vi "usrp_mimo_ofdm_2x2_freq_MRC.vi"() -> ()   [LabVIEW 2014]
uses:
  <instrlib>/niUSRP/niUSRP Timestamp.ctl
  <vilib>/addons/Modulation/Analog/controls/Complex Data Waveform.ctl
  <vilib>/addons/Modulation/Digital/General/MT Generate Bits (Galois, PN Order).vi
  <vilib>/addons/Modulation/Digital/Support/Common/Validators/mod_Generate Bits Validate.vi
  <vilib>/addons/Modulation/Analog/support/mod_Set Error Source.vi
  <instrlib>/niUSRP/niUSRP Configure Time Start Trigger.vi
  <vilib>/addons/Modulation/Digital/General/MT Generate QAM System Parameters(M).vi
  <vilib>/addons/Modulation/Digital/Support/Common/Validators/mod_Generate Filter Coefficients Validate.vi
  <vilib>/addons/Modulation/Digital/General/subVIs/mod_Generate Filter Coefficients.vi
  <vilib>/addons/Modulation/Digital/General/subVIs/mod_Generate Bits PN Sequence.vi
  <vilib>/addons/Modulation/Digital/General/MT Map Bits to QAM Symbols.vi
  <vilib>/addons/Modulation/Digital/General/MT Apply Pulse Shaping Filter (Generic).vi
  <instrlib>/niUSRP/niUSRP Write Tx Data (2D CDB).vi
  <instrlib>/niUSRP/niUSRP Fetch Rx Data (2D CDB).vi
  <vilib>/addons/Modulation/Digital/General/MT Apply Matched Filter (Generic).vi
  <vilib>/addons/Modulation/Digital/General/MT Align to Ideal Symbols (Generic).vi
  <vilib>/measure/maspectr.llb/FFT Power Spectrum and PSD for 1 Chan (CDB).vi
  <vilib>/addons/Modulation/Digital/General/MT Map QAM Symbols to Bits.vi
  <vilib>/addons/Modulation/niDMT.lvlib
  <vilib>/measure/NI_MAPro.lvlib
  <vilib>/addons/Modulation/niAMT.lvlib
panel:
  out "Decoded Constellation Map":cdb[](graph)
  out "Decoded Constellation Map 2":cdb[](graph)
  out "Waveform Chart":i16(graph)
  out "sum":i16
  out "x = 0?":bool
  out "input bits stream":i8[](array[numeric]) caption="input bit stream"
  out "output bit stream":i8[](array[numeric])
  in  "CP length":u32=32 caption="CP Size"
  in  "Message Carrier":u32=128
  in  "FFT Size":u32=256
  in  "RXa:Timebase Clock Source":string(combo)="Internal"
  in  "RXa:Reference Frequency Source":string(combo)="Internal"
  in  "TXa:Timebase Clock Source":string(combo)="Internal"
  in  "TXa:Reference Frequency Source":string(combo)="Internal"
  out "OFF":bool=TRUE
  out "RX error":bool
  out "TX error":bool
  out "ERROR":bool
  out "Decoded Constellation Map 1":cdb[](graph)
  in  "TX timeout":dbl=10.0
  out "error IO":errorcluster
  in  "stop":bool
  out "Transmitted Constellation Map":cluster{dbl[], dbl[]}[](graph)
  out "PSD of Received Signal":cluster{"f0":dbl, "df":dbl, "magnitude":dbl[]}[](graph)
  out "USRP timestamp":T1={"whole seconds"=11, "fractional seconds"=0.9000012199999999}
  in  "number of samples":i64=100000
  in  "M-QAM (16)":i32=16
  in  "total bits (128)":i32=512 caption="total bits (512)"
  in  "filter length (symbols)":i32=8
  in  "filter parameter":dbl=0.5 format="%.2f"
  in  "samples per symbol (16)":i32=4
  in  "pulse shaping filter (none)":T2(ring)=enum."Raised Cosine"
  in  "RXb:Timebase Clock Source":string(combo)="Mimo"
  in  "RXb:Reference Frequency Source":string(combo)="Mimo"
  in  "TXb:Timebase Clock Source":string(combo)="Mimo"
  in  "TXb:Reference Frequency Source":string(combo)="Mimo"
  in  "RXb Active Antenna":string="RX2"
  in  "TXb Active Antenna":string="TX1"
  in  "RXb Gain":dbl
  in  "TXb Gain":dbl
  in  "RXa Active Antenna":string="RX2"
  in  "RXa Gain":dbl
  in  "TXa Active Antenna":string="TX1"
  in  "TXa Gain":dbl
  in  "Carrier Frequency":dbl=1200000000.0 format="%#_6p"
  in  "IQ Rate":dbl=1000000.0 format="%#_6p"
  in  "TX device names":refnum<k15>="192.168.10.2;192.168.10.5"
  in  "start trigger time":T1={"whole seconds"=4, "fractional seconds"=0.1}
  in  "RX device names":refnum<k15>="192.168.10.2;192.168.10.5"
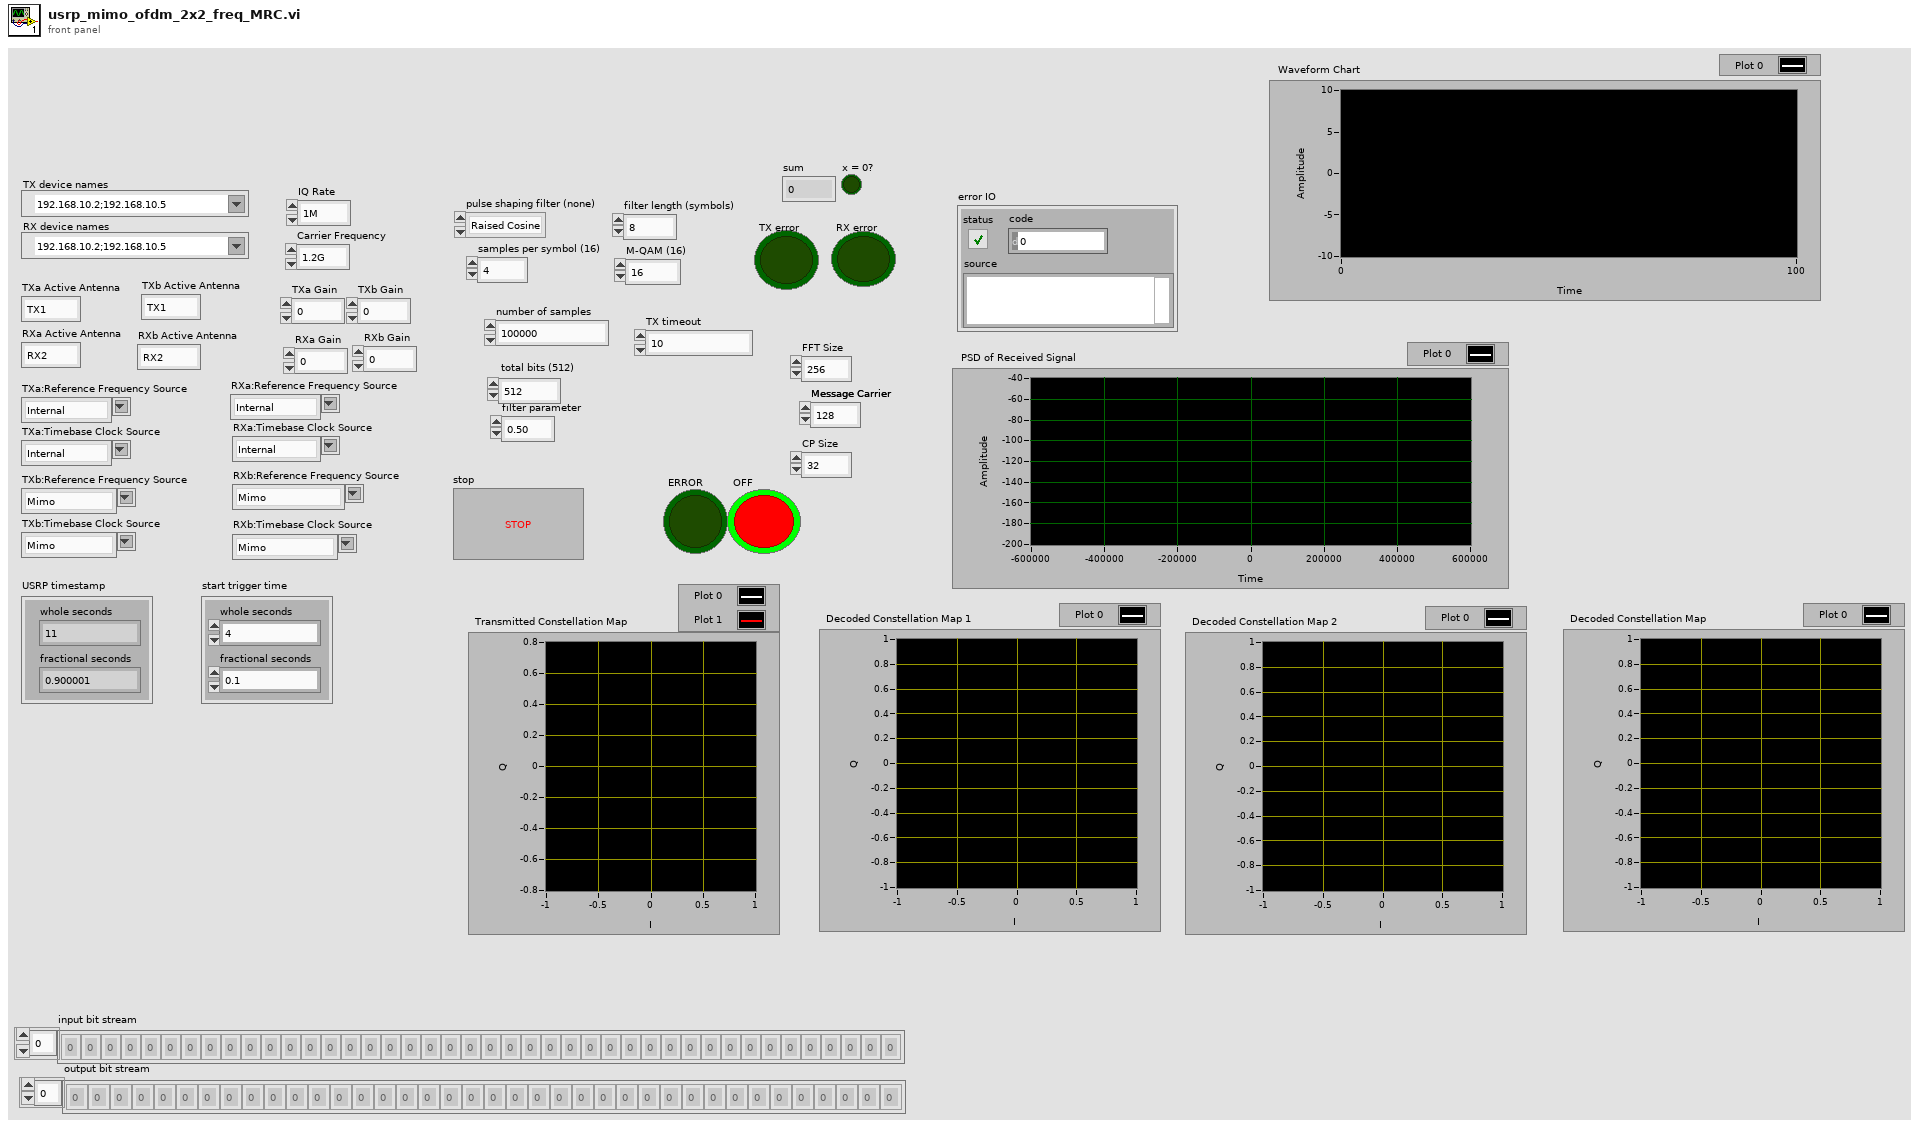
[diagram p1: front panel]
types:
  T1 = typedef "niUSRP Timestamp.ctl" = cluster{"whole seconds":u64, "fractional seconds":dbl}
  T2 = enum16{"none", "Raised Cosine", "Root Raised Cos", "Gaussian"}
  T3 = enum16{"FSK", "PSK", "QAM", "MSK", "PAM", "ASK", "CPM"}
  T4 = cluster{"samples per symbol (16)":i32, "symbol map":cdb[]}
  T5 = typedef "niAMT.lvlib/Complex Data Waveform.ctl" = cluster{"t0":dbl, "dt":dbl, "Y":cdb[]}
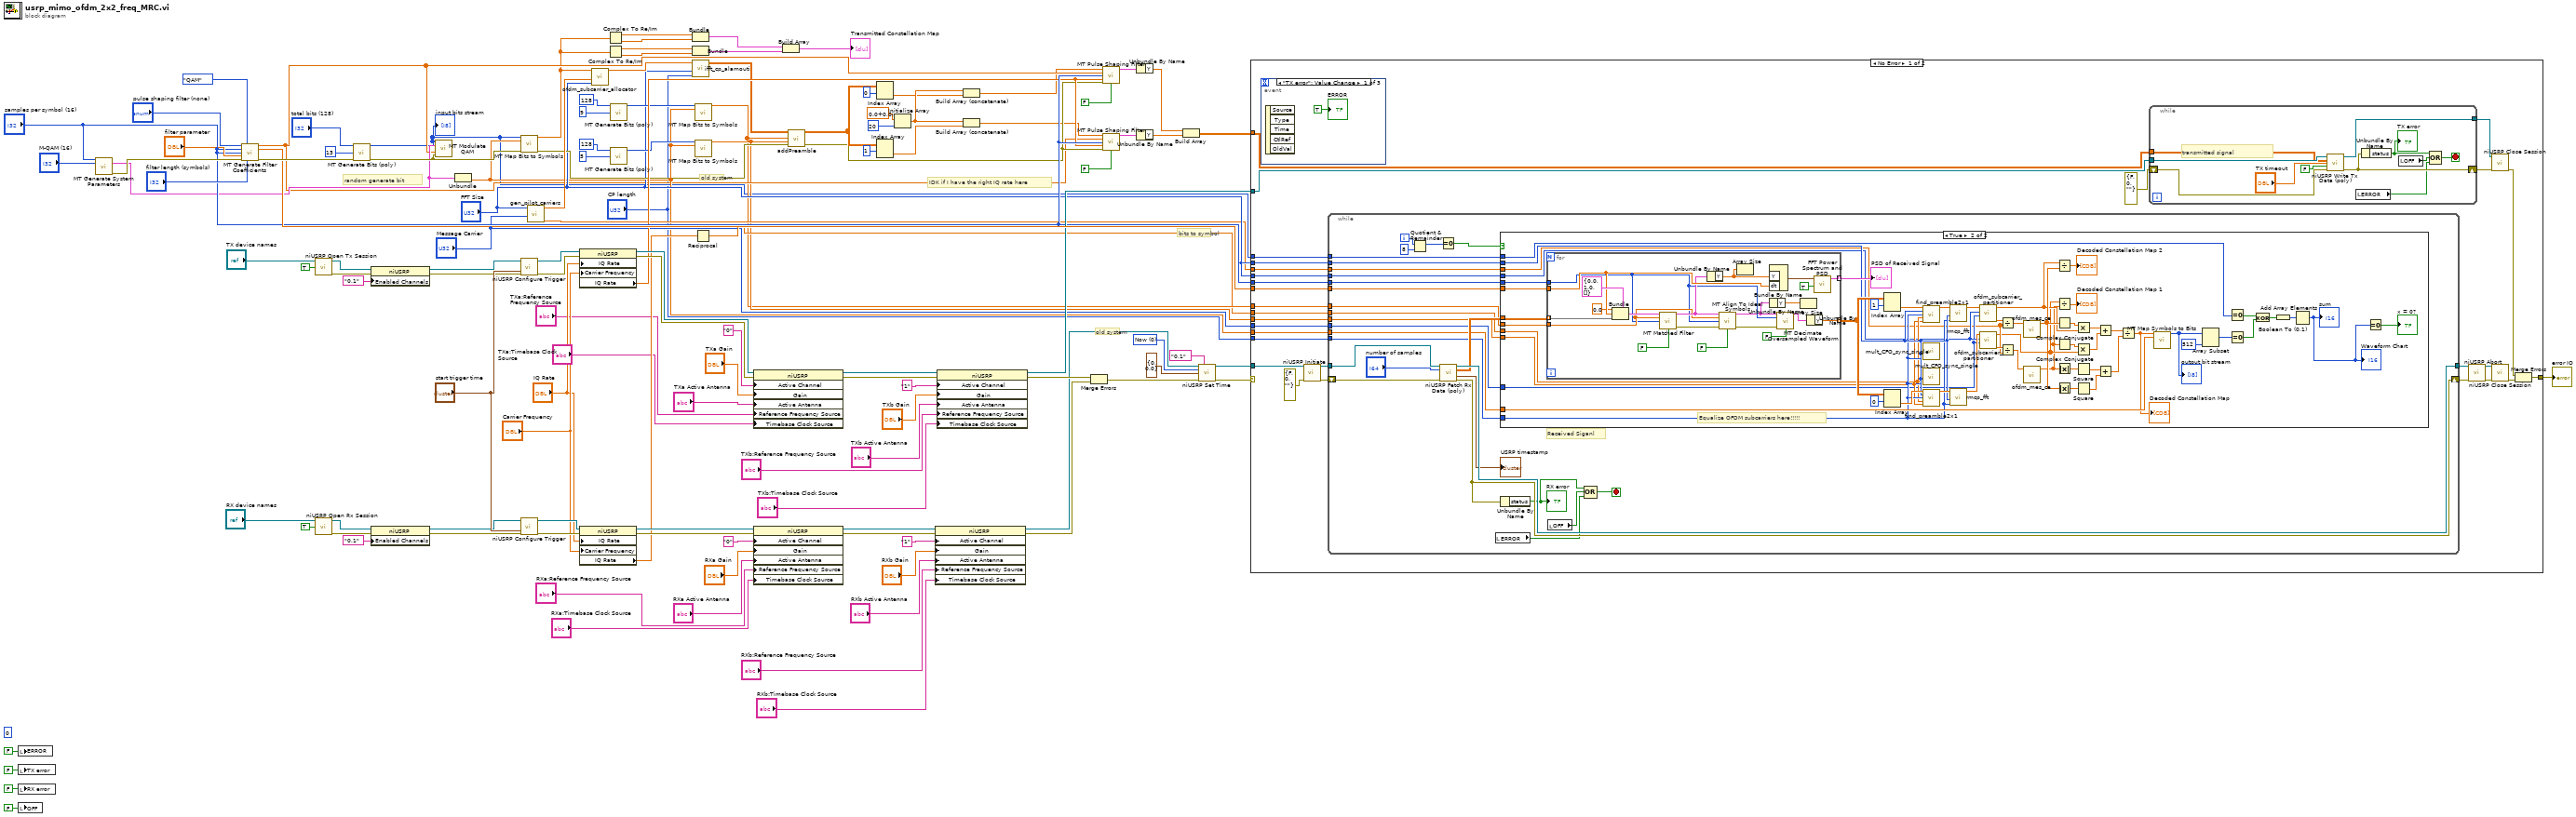
[diagram p0: block diagram]
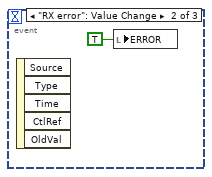
[diagram p2: hidden frame]
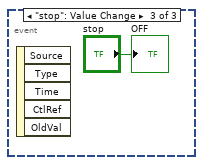
[diagram p3: hidden frame]
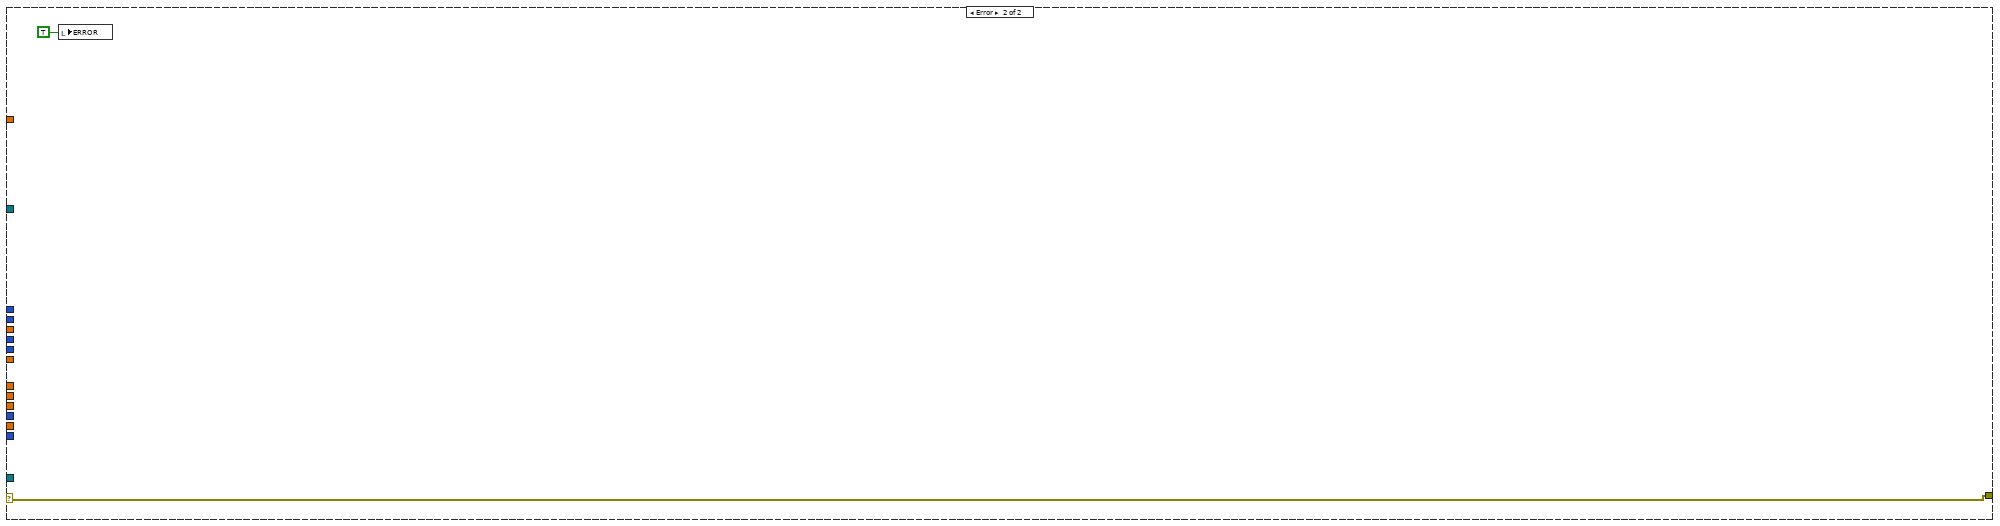
[diagram p5: hidden frame]
diagram:
  (unwired) 0 ("index")
  w84 = 0 items=["Now", "Next Timebase Edge"] ("apply timestamp")
  # "IDK if I have the right IQ rate here"
  # "bits to symbol"
  # "old system"
  # "old system"
  # "random generate bit"
  n1 = local write "ERROR"(FALSE) -> ()
  n2 = local write "TX error"(FALSE) -> ()
  n3 = local write "RX error"(FALSE) -> ()
  n4 = local write "OFF"(FALSE) -> ()
  n5 = call-poly <vilib>:"MT Generate System Parameters.vi"("samples per symbol (16)"="samples per symbol (16)", "M-QAM (16)"="M-QAM (16)") -> ("QAM system parameters"=w26:T4, "error out"=w74:errorcluster)  [unwired: 11 in, 1 out]
  n6 = call <vilib>:"MT Generate Filter Coefficients.vi"("pulse shaping filter (none)"="pulse shaping filter (none)", "modulation type"=T3."QAM", "pulse shaping samples per symbol (16)"="samples per symbol (16)", "matched samples per symbol (16)"="samples per symbol (16)", "filter parameter"="filter parameter", "error in (no error)"=w74, "filter length (symbols)"="filter length (symbols)") -> ("pulse shaping filter coefficients"=w17:dbl[], "matched filter coefficients"=w52:dbl[], "error out"=w73:errorcluster)  [unwired: 6 in]
  n7 = call <instrlib>:"niUSRP Open Tx Session.vi"("device names"="TX device names", "reset"=TRUE) -> ("session handle out"=w57:refnum<k15>, "error out"=w56:errorcluster)  [unwired: 12 in]
  n8 = call <instrlib>:"niUSRP Open Rx Session.vi"("device names"="RX device names", "reset"=TRUE) -> ("session handle out"=w59:refnum<k15>, "error out"=w58:errorcluster)  [unwired: 12 in]
  n9 = call-poly <vilib>:"MT Generate Bits (poly).vi"("total bits (128)"="total bits (128)", "PN sequence order (9)"=13, "error in (no error)"=w73) -> ("output bit stream"=w13:i8[], "error out"=w43:errorcluster)  [unwired: 10 in, 1 out]
  "input bits stream" <- w13
  n10 = property class="niUSRP"(reference=w57, error in=w56, "Enabled Channels"="0,1" ("Configuration:Enabled Channels")) -> (reference out=w118:refnum<k15>, error out=w117:errorcluster)
  n11 = property class="niUSRP"(reference=w59, error in=w58, "Enabled Channels"="0,1" ("Configuration:Enabled Channels")) -> (reference out=w116:refnum<k15>, error out=w115:errorcluster)
  n12 = call <vilib>:"MT Modulate QAM.vi"("input bit stream"=w13, "QAM system parameters"=w26, "pulse shaping filter coefficients"=w17, "error in (no error)"=w43) -> ()  [unwired: 9 in, 3 out]
  n13 = Unbundle(w26) -> ("symbol map"=w20:cdb[])  [unwired: 1 out]
  n14 = call-poly <instrlib>:"niUSRP Configure Trigger.vi"("session handle"=w118, "start trigger time"="start trigger time", "error in (no error)"=w117) -> ("session handle out"=w110:refnum<k15>, "error out"=w109:errorcluster)  [unwired: 11 in]
  n15 = call-poly <instrlib>:"niUSRP Configure Trigger.vi"("session handle"=w116, "start trigger time"="start trigger time", "error in (no error)"=w115) -> ("session handle out"=w114:refnum<k15>, "error out"=w113:errorcluster)  [unwired: 11 in]
  n16 = call-poly <vilib>:"MT Map Bits to Symbols.vi"("input bit stream"=w13, "symbol map"=w20, "error in (no error)"=w43) -> ("symbols"=w14:cdb[], "error out"=w30:errorcluster)  [unwired: 11 in]
  n17 = call "gen_pilot_carriers.vi"("message carrier"="Message Carrier", "FFT size"="FFT Size") -> ("RX pilot carriers"=w21:cdb[], "TX pilot carriers"=w42:cdb[])  [unwired: 8 in]
  n18 = property class="niUSRP"(reference=w110, error in=w109, "IQ Rate"="IQ Rate", "Carrier Frequency"="Carrier Frequency") -> (reference out=w106:refnum<k15>, error out=w105:errorcluster, "IQ Rate"=w37:dbl)
  n19 = property class="niUSRP"(reference=w114, error in=w113, "IQ Rate"="IQ Rate", "Carrier Frequency"="Carrier Frequency") -> (reference out=w112:refnum<k15>, error out=w111:errorcluster, "IQ Rate"=w69:dbl)
  n20 = call "ofdm_subcarrier_allocator.vi"("fft size"="FFT Size", "pilot symbol"=w42, "message symbol"=w14) -> ("OFDM symbol"=w41:cdb[])  [unwired: 8 in]
  n21 = Complex To Re/Im(x + iy=w14) -> (x=w67:dbl[], y=w66:dbl[])
  n22 = Complex To Re/Im(x + iy=w14) -> (x=w65:dbl[], y=w64:dbl[])
  n23 = call-poly <vilib>:"MT Generate Bits (poly).vi"("total bits (128)"=128, "PN sequence order (9)"=9) -> ("output bit stream"=w23:i8[])  [unwired: 11 in, 2 out]
  n24 = call-poly <vilib>:"MT Generate Bits (poly).vi"("total bits (128)"=128, "PN sequence order (9)"=5) -> ("output bit stream"=w25:i8[])  [unwired: 11 in, 2 out]
  n25 = Bundle(w67, w66) -> (w62:cluster{dbl[], dbl[]})  [unwired: 1 in]
  n26 = Bundle(w65, w64) -> (w63:cluster{dbl[], dbl[]})  [unwired: 1 in]
  n27 = call "ifft_cp_alamouti.vi"("CP Length"="CP length", "FFT Size"="FFT Size", "Modulated Stream"=w41) -> ("Baseband Streams"=w32:cdb[][])  [unwired: 8 in]
  n28 = call-poly <vilib>:"MT Map Bits to Symbols.vi"("input bit stream"=w23, "symbol map"=w20) -> ("symbols"=w15:cdb[])  [unwired: 12 in, 1 out]
  n29 = call-poly <vilib>:"MT Map Bits to Symbols.vi"("input bit stream"=w25, "symbol map"=w20) -> ("symbols"=w16:cdb[])  [unwired: 12 in, 1 out]
  n30 = Reciprocal(x=w69) -> (1/x=w68:dbl)
  n31 = property class="niUSRP"(reference=w106, error in=w105, "Active Channel"="0", "Gain"="TXa Gain", "Active Antenna"="TXa Active Antenna", "Reference Frequency Source"="TXa:Reference Frequency Source", "Timebase Clock Source"="TXa:Timebase Clock Source") -> (reference out=w96:refnum<k15>, error out=w95:errorcluster)
  n32 = property class="niUSRP"(reference=w112, error in=w111, "Active Channel"="0", "Gain"="RXa Gain", "Active Antenna"="RXa Active Antenna", "Reference Frequency Source"="RXa:Reference Frequency Source", "Timebase Clock Source"="RXa:Timebase Clock Source") -> (reference out=w98:refnum<k15>, error out=w97:errorcluster)
  n33 = Build Array(w62, w63) -> (→"Transmitted Constellation Map":cluster{dbl[], dbl[]}[])
  n34 = call "addPreamble.vi"("Input Symbol Stream"=w32, "Training Sequence"=w15, "Training Sequence 2"=w16, "error in (no error)"=w30) -> ("Output Transmit \nPackets"=w31:cdb[][], "error out"=w29:errorcluster)  [unwired: 10 in]
  n35 = Index Array(array=w31, index (row)=0) -> (element=w1:cdb[])  [unwired: 1 in]
  n36 = Index Array(array=w31, index (row)=1) -> (element=w2:cdb[])  [unwired: 1 in]
  n37 = Initialize Array(cdb 0.0+0.0i ("element"), 20 ("dimension size")) -> (w3:cdb[])
  n38 = property class="niUSRP"(reference=w98, error in=w97, "Active Channel"="1", "Gain"="RXb Gain", "Active Antenna"="RXb Active Antenna", "Reference Frequency Source"="RXb:Reference Frequency Source", "Timebase Clock Source"="RXb:Timebase Clock Source") -> (reference out=w54:refnum<k15>, error out=w82:errorcluster)
  n39 = property class="niUSRP"(reference=w96, error in=w95, "Active Channel"="1", "Gain"="TXb Gain", "Active Antenna"="TXb Active Antenna", "Reference Frequency Source"="TXb:Reference Frequency Source", "Timebase Clock Source"="TXb:Timebase Clock Source") -> (reference out=w55:refnum<k15>, error out=w81:errorcluster)
  n40 = Build Array (concatenate)(w3, w1) -> (w5:cdb[])
  n41 = Build Array (concatenate)(w3, w2) -> (w4:cdb[])
  n42 = Merge Errors(w81, w82) -> (w80:errorcluster)
  n43 = call-poly <vilib>:"MT Pulse Shaping Filter.vi"("symbols"=w5, "pulse shaping filter coefficients"=w17, "samples per symbol (16)"="samples per symbol (16)", "symbol rate (Hz)"=w37, "error in (no error)"=w29, "reset? (T)"=FALSE) -> ("output complex waveform"=w35:T5)  [unwired: 8 in, 1 out]
  n44 = call-poly <vilib>:"MT Pulse Shaping Filter.vi"("symbols"=w4, "pulse shaping filter coefficients"=w17, "samples per symbol (16)"="samples per symbol (16)", "symbol rate (Hz)"=w37, "error in (no error)"=w29, "reset? (T)"=FALSE) -> ("output complex waveform"=w34:T5)  [unwired: 8 in, 1 out]
  n45 = Unbundle By Name(w35) -> ("Y"=w8:cdb[])
  n46 = Unbundle By Name(w34) -> ("Y"=w33:cdb[])
  n47 = Build Array(w8, w33) -> (w11:cdb[][])
  n48 = call <instrlib>:"niUSRP Set Time.vi"("session handle"=w54, "channel list"="0,1" ("Configuration:Enabled Channels"), "apply timestamp"=w84, "timestamp"=T1 {"whole seconds"=0, "fractional seconds"=0.0}, "error in (no error)"=w80) -> ("session handle out"=w53:refnum<k15>, "error out"=w79:errorcluster)  [unwired: 9 in]
  n49 = case shown="No Error" w79 {
    selector: w79 -> [_ w270]
    tunnel: w53 -> [w139 _]
    tunnel: w55 -> [w152 _]
    tunnel: w11 -> [w153 _]
    tunnel: w68 -> [w143 _]
    tunnel: [w140 w270] -> w61
    tunnel: w52 -> [w136 _]
    tunnel: "samples per symbol (16)" -> [w135 _]
    tunnel: "FFT Size" -> [w134 _]
    tunnel: "Message Carrier" -> [w133 _]
    tunnel: w15 -> [w132 _]
    tunnel: w16 -> [w131 _]
    tunnel: "FFT Size" -> [w130 _]
    tunnel: "CP length" -> [w129 _]
    tunnel: w21 -> [w128 _]
    tunnel: w20 -> [w127 _]
    tunnel: w13 -> [w126 _]
    frame No Error {
      n50 = event shown="[0] \"TX error\": Value Change" {
        selector: _ -> [_ _ _]
        dyn-events: _ -> [_ _ _]
        timeout: _ -> [_ _ _]
        event "TX error": Value Change {
          n51 = event-data() -> ()  [unwired: 1 in, 5 out]
          "ERROR" <- TRUE
        }
        event "RX error": Value Change {
          n52 = event-data() -> ()  [unwired: 1 in, 5 out]
          n53 = local write "ERROR"(TRUE) -> ()
        }
        event "stop": Value Change {
          n54 = event-data() -> ()  [unwired: 1 in, 5 out]
          "OFF" <- "stop"
        }
      }
      n55 = call <instrlib>:"niUSRP Initiate.vi"("session handle"=w139, "error in (no error)"=errorcluster {"status"=FALSE, "code"=0, "source"=""}) -> ("session handle out"=w151:refnum<k15>, "error out"=w150:errorcluster)  [unwired: 12 in]
      n56 = while {
        tunnel: w151 -> [w182]
        shift-right: [w176] -> w149
        shift-left: w150 -> [w181]
        tunnel: [w180] -> w148
        tunnel: w143 -> [w177]
        tunnel: w136 -> [w173]
        tunnel: w135 -> [w172]
        tunnel: w134 -> [w169]
        tunnel: w133 -> [w168]
        tunnel: w132 -> [w167]
        tunnel: w131 -> [w166]
        tunnel: w130 -> [w165]
        tunnel: w129 -> [w164]
        tunnel: w128 -> [w163]
        tunnel: w127 -> [w162]
        tunnel: w126 -> [w161]
        i -> [w160]
        stop <- w174 stop-if-true
        # "Received Siganl"
        n57 = Quotient & Remainder(x=w160, y=8) -> (x-y*floor(x/y)=w158:i32)  [unwired: 1 out]
        n58 = Equal To 0?(x=w158) -> (x = 0?=w157:bool)
        n59 = call-poly <instrlib>:"niUSRP Fetch Rx Data (poly).vi"("session handle"=w182, "number of samples"="number of samples", "error in (no error)"=w181) -> ("session handle out"=w180:refnum<k15>, "data"=w178:cdb[][], "timestamp"=→"USRP timestamp":T1, "error out"=w176:errorcluster)  [unwired: 9 in]
        n60 = local read "ERROR"() -> (w171:bool)
        n61 = case shown="True" w157 {
          tunnel: w178 -> [_ w234]
          tunnel: w177 -> [_ w236]
          tunnel: w173 -> [_ w233]
          tunnel: w172 -> [_ w232]
          tunnel: w169 -> [_ w202]
          tunnel: w168 -> [_ w201]
          tunnel: w167 -> [_ w204]
          tunnel: w166 -> [_ w203]
          tunnel: w165 -> [_ w206]
          tunnel: w164 -> [_ w205]
          tunnel: w163 -> [_ w200]
          tunnel: w162 -> [_ w231]
          tunnel: w161 -> [_ w223]
          frame False {
          }
          frame True {
            # "Equalize OFDM subcarriers here!!!!!"
            n62 = for {
              tunnel: w236 -> [w253]
              tunnel: [w255] -> w235 mode=indexing
              tunnel: w234 -> [w252] mode=indexing
              tunnel: w233 -> [w248]
              tunnel: w232 -> [w245]
              tunnel: [w237] -> w210 mode=indexing
              n63 = Bundle(cluster=T5 {"t0"=0.0, "dt"=1.0, "Y"=[]} ("input complex waveform"), "t0"=0.0, "dt"=w253, "Y"=w252) -> (w250:T5)
              n64 = call-poly <vilib>:"MT Matched Filter.vi"("input complex waveform"=w250, "matched filter coefficients"=w248, "samples per symbol (16)"=w245, "reset? (T)"=FALSE) -> ("output complex waveform"=w249:T5, "error out"=w247:errorcluster)  [unwired: 10 in]
              n65 = Unbundle By Name(w249) -> ("Y"=w240:cdb[])
              n66 = call-poly <vilib>:"MT Align To Ideal Symbols.vi"("input complex waveform"=w249, "matched filter coefficients"=w248, "samples per symbol (16)"=w245, "error in (no error)"=w247, "reset? (T)"=FALSE) -> ("output complex waveform"=w239:T5, "error out"=w246:errorcluster)  [unwired: 8 in, 1 out]
              n67 = Array Size(array=w240) -> ()  [unwired: 1 out]
              n68 = Bundle By Name("Y"=w240, "dt"=w253) -> (w257:waveform(cdb))  [unwired: 1 in]
              n69 = Unbundle By Name(w239) -> ("Y"=w238:cdb[])
              n70 = call <vilib>:"MT Decimate Oversampled Waveform.vi"("input complex waveform"=w239, "decimation factor"=w245, "error in (no error)"=w246, "reset? (T)"=FALSE) -> ("output complex waveform"=w244:T5)  [unwired: 10 in, 1 out]
              n71 = Array Size(array=w238) -> ()  [unwired: 1 out]
              n72 = Unbundle By Name(w244) -> ("Y"=w237:cdb[])
              n73 = call-poly <vilib>:"FFT Power Spectrum and PSD.vi"("dB On (F)"=TRUE, "time signal"=w257) -> ("Power Spectrum / PSD"=w255:cluster{"f0":dbl, "df":dbl, "magnitude":dbl[]})  [unwired: 6 in, 3 out]
            }
            "PSD of Received Signal" <- w235
            n74 = Index Array(array=w210, index (row)=1) -> (element=w207:cdb[])  [unwired: 1 in]
            n75 = Index Array(array=w210, index (row)=0) -> (element=w208:cdb[])  [unwired: 1 in]
            n76 = call "find_preamble2x1.vi"("received \ntime symbol"=w207, "FFT Size"=w206, "CP Length"=w205, "1st preamble"=w204, "2nd preamble"=w203) -> ("OFDM Symbol"=w212:cdb[])  [unwired: 10 in]
            n77 = call "mult_CFO_sync_single.vi"("CP length"=w205, "FFT size"=w206) -> ()  [unwired: 9 in, 1 out]
            n78 = call "mult_CFO_sync_single.vi"("CP length"=w205, "FFT size"=w206) -> ()  [unwired: 9 in, 1 out]
            n79 = call "find_preamble2x1.vi"("received \ntime symbol"=w208, "FFT Size"=w206, "CP Length"=w205, "1st preamble"=w204, "2nd preamble"=w203) -> ("OFDM Symbol"=w217:cdb[])  [unwired: 10 in]
            n80 = call "rmcp_fft.vi"("CP length"=w205, "fft size"=w206, "time symbol"=w212) -> ("freq output"=w213:cdb[])  [unwired: 8 in]
            n81 = call "rmcp_fft.vi"("CP length"=w205, "fft size"=w206, "time symbol"=w217) -> ("freq output"=w225:cdb[])  [unwired: 8 in]
            n82 = call "ofdm_subcarrier_partitioner.vi"("message carrier"=w201, "FFT size"=w202, "received symbol"=w213) -> ("pilot subcarriers"=w215:cdb[], "message subcarriers"=w187:cdb[])  [unwired: 7 in]
            n83 = call "ofdm_subcarrier_partitioner.vi"("message carrier"=w201, "FFT size"=w202, "received symbol"=w225) -> ("pilot subcarriers"=w227:cdb[], "message subcarriers"=w186:cdb[])  [unwired: 7 in]
            n84 = Divide(x=w215, y=w200) -> (x/y=w214:cdb[])
            n85 = Divide(x=w227, y=w200) -> (x/y=w226:cdb[])
            n86 = call "ofdm_mes_ce.vi"("ZF \nchannel \nestimates"=w214) -> ("interpolated\n mes carrier CE"=w188:cdb[])  [unwired: 10 in]
            n87 = call "ofdm_mes_ce.vi"("ZF \nchannel \nestimates"=w226) -> ("interpolated\n mes carrier CE"=w185:cdb[])  [unwired: 10 in]
            n88 = Divide(x=w187, y=w188) -> (x/y=→"Decoded Constellation Map 2":cdb[])
            n89 = Divide(x=w186, y=w185) -> (x/y=→"Decoded Constellation Map 1":cdb[])
            n90 = Complex Conjugate(1:w188) -> (0:w194:cdb[])
            n91 = Complex Conjugate(1:w185) -> (0:w193:cdb[])
            n92 = Absolute Value(x=w185) -> (abs(x)=w198:dbl[])
            n93 = Absolute Value(x=w188) -> (abs(x)=w197:dbl[])
            n94 = Multiply(x=w194, y=w187) -> (x*y=w192:cdb[])
            n95 = Multiply(x=w193, y=w186) -> (x*y=w191:cdb[])
            n96 = Square(x=w198) -> (x^2=w196:dbl[])
            n97 = Square(x=w197) -> (x^2=w195:dbl[])
            n98 = Add(x=w192, y=w191) -> (x+y=w190:cdb[])
            n99 = Add(x=w196, y=w195) -> (x+y=w189:dbl[])
            n100 = Divide(x=w190, y=w189) -> (x/y=w184:cdb[])
            "Decoded Constellation Map" <- w184
            n101 = call-poly <vilib>:"MT Map Symbols to Bits.vi"("symbols"=w184, "symbol map"=w231) -> ("output bit stream"=w229:i8[])  [unwired: 12 in, 1 out]
            "output bit stream" <- w229
            n102 = Array Subset(array=w229, length=512) -> (w221:i8[])  [unwired: 1 in]
            n103 = Equal To 0?(x=w223) -> (x = 0?=w220:bool[])
            n104 = Equal To 0?(x=w221) -> (x = 0?=w222:bool[])
            n105 = Exclusive Or(1:w222, 2:w220) -> (0:w219:bool[])
            n106 = Boolean To (0,1)(Boolean=w219) -> (0, 1=w218:i16[])
            n107 = Add Array Elements(numeric array=w218) -> (sum=w216:i16)
            "sum" <- w216
            "Waveform Chart" <- w216
            n108 = Equal To 0?(x=w216) -> (x = 0?=→"x = 0?":bool)
          }
        }
        n109 = Unbundle By Name(w176) -> ("status"=w175:bool)
        "RX error" <- w175
        n110 = local read "OFF"() -> (w170:bool)
        n111 = Compound Arithmetic op=OR(w175, w170, w171) -> (w174:bool)
      }
      n112 = while {
        tunnel: w153 -> [w264]
        tunnel: w152 -> [w268]
        tunnel: [w267] -> w145
        shift-right: [w263] -> w144
        shift-left: errorcluster {"status"=FALSE, "code"=0, "source"=""} ("error out") -> [w266]
        stop <- w261 stop-if-true
        # "transmitted signal"
        n113 = call-poly <instrlib>:"niUSRP Write Tx Data (poly).vi"("session handle"=w268, "data"=w264, "timeout"="TX timeout", "end of data?"=FALSE, "error in (no error)"=w266) -> ("session handle out"=w267:refnum<k15>, "error out"=w263:errorcluster)  [unwired: 9 in]
        n114 = local read "ERROR"() -> (w259:bool)
        n115 = Unbundle By Name(w263) -> ("status"=w262:bool)
        "TX error" <- w262
        n116 = local read "OFF"() -> (w258:bool)
        n117 = Compound Arithmetic op=OR(w262, w258, w259) -> (w261:bool)
      }
      n118 = call <instrlib>:"niUSRP Abort.vi"("session handle"=w148, "error in (no error)"=w149) -> ("session handle out"=w147:refnum<k15>, "error out"=w146:errorcluster)  [unwired: 12 in]
      n119 = call <instrlib>:"niUSRP Close Session.vi"("session handle"=w145, "error in (no error)"=w144) -> ("error out"=w141:errorcluster)  [unwired: 13 in]
      n120 = call <instrlib>:"niUSRP Close Session.vi"("session handle"=w147, "error in (no error)"=w146) -> ("error out"=w142:errorcluster)  [unwired: 13 in]
      n121 = Merge Errors(w141, w142) -> (w140:errorcluster)
    }
    frame Error {
      n122 = local write "ERROR"(TRUE) -> ()
    }
  }
  "error IO" <- w61
